vi "Quaternary_Layer.vi"(2 "Debug Mode":bool, 3 "Elapsed Time (s)":dbl, 4 "State":enum16{"Edit", "Start", "Run", "End", "Idle"}(ring), 5 "Argument List In":string[](array[string])) -> (0 "Status Out":string, 1 "Argument List Out":string[](array[string]))   [LabVIEW 2011]
panel:
  in  "PH3 run":bool
  in  "AsH3 run":bool
  in  "In run":bool
  in  "Ga run":bool
  in  "PH3 Flow":dbl
  in  "AsH3 Flow":dbl
  in  "In Flow":dbl
  in  "Ga Flow":dbl
  in  "Cancel":bool
  in  "OK":bool
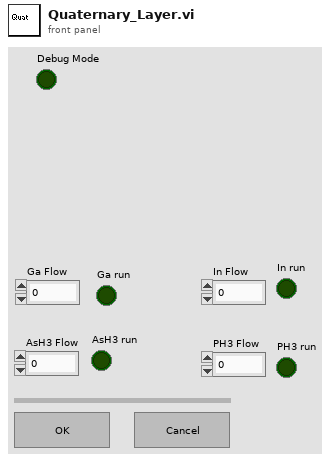
[diagram p1: front panel]
types:
  T1 = enum16{"Discrete", "Continuous", "Instantaneous"}
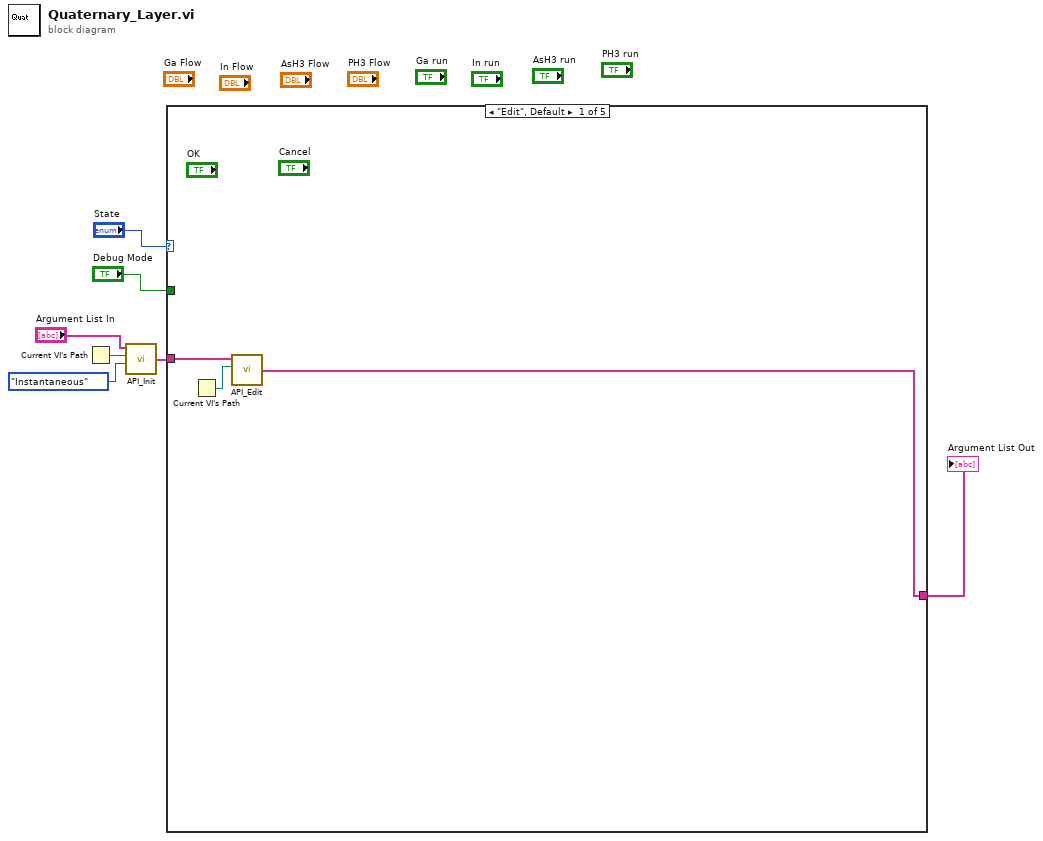
[diagram p0: block diagram]
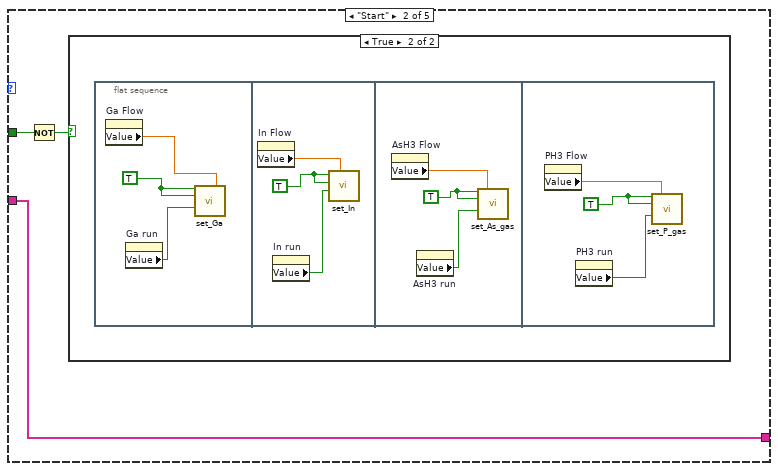
[diagram p2: hidden frame]
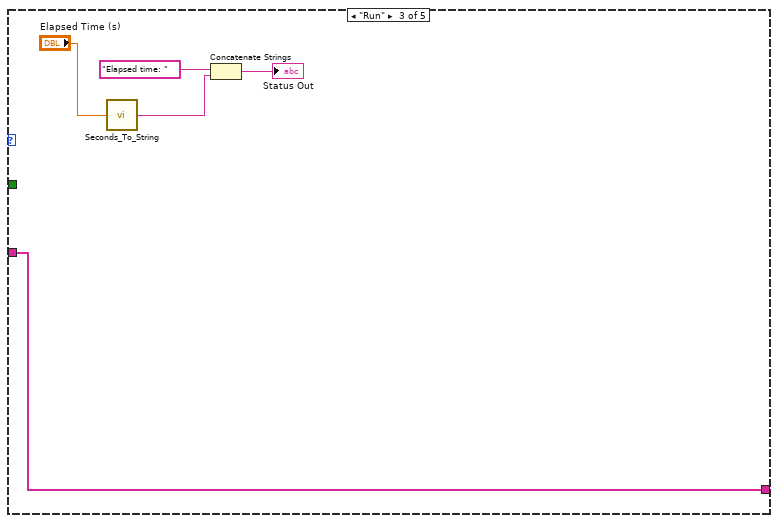
[diagram p4: hidden frame]
diagram:
  n1 = Current VI's Path() -> (path=w4:path)
  n2 = call "API_Init.vi"("API Mode"=T1."Instantaneous", "VI Path"=w4, "Argument List In"="Argument List In") -> ("Argument List Out"=w3:string[])  [unwired: 1 in]
  n3 = case shown="\"Edit\", Default" "State" {
    tunnel: [w8 w13 w26 w31 w32] -> w6
    tunnel: w3 -> [w9 w13 w26 w31 w32]
    tunnel: "Debug Mode" -> [_ w12 _ _ _]
    frame "Edit", Default {
      n4 = Current VI's Path() -> (path=w10:path)
      n5 = call "API_Edit.vi"("VI Path"=w10, "Argument List In"=w9) -> ("Argument List Out"=w8:string[])  [unwired: 2 in]
    }
    frame "Start" {
      n6 = Not(x=w12) -> (.not. x?=w11:bool)
      n7 = case shown="True" w11 {
        frame False {
        }
        frame True {
          n8 = flat-sequence {
            frame #0 {
              w16 = TRUE ("Ga Active")
              n9 = property on="Ga Flow" class="DigNum (strict)"() -> ("Value"=w15:dbl)  [unwired: 2 in, 2 out]
              n10 = property on="Ga run" class="Bool (strict)"() -> ("Value"=w14:bool)  [unwired: 2 in, 2 out]
              n11 = call "set_Ga.vi"("Ga Active"=w16, "Ga Flow 1"=w15, "Ga Bubbler"=w16, "Ga Run"=w14) -> ()  [unwired: 4 in, 8 out]
            }
            frame #1 {
              w19 = TRUE ("Ga Active")
              n12 = property on="In Flow" class="DigNum (strict)"() -> ("Value"=w18:dbl)  [unwired: 2 in, 2 out]
              n13 = property on="In run" class="Bool (strict)"() -> ("Value"=w17:bool)  [unwired: 2 in, 2 out]
              n14 = call "set_In.vi"("Indium Flow"=w18, "In Run"=w17, "In Bubbler"=w19, "In Active"=w19) -> ()  [unwired: 1 in, 5 out]
            }
            frame #2 {
              w21 = TRUE ("Ga Active")
              n15 = property on="AsH3 Flow" class="DigNum (strict)"() -> ("Value"=w22:dbl)  [unwired: 2 in, 2 out]
              n16 = property on="AsH3 run" class="Bool (strict)"() -> ("Value"=w20:bool)  [unwired: 2 in, 2 out]
              n17 = call "set_As_gas.vi"("As_Gas Active"=w21, "As_Gas Flow"=w22, "As_Gas In"=w21, "As_Gas Run"=w20) -> ()  [unwired: 2 in, 10 out]
            }
            frame #3 {
              w25 = TRUE ("Ga Active")
              n18 = property on="PH3 Flow" class="DigNum (strict)"() -> ("Value"=w24:dbl)  [unwired: 2 in, 2 out]
              n19 = property on="PH3 run" class="Bool (strict)"() -> ("Value"=w23:bool)  [unwired: 2 in, 2 out]
              n20 = call "set_P_gas.vi"("P_Gas Active"=w25, "P_Gas Flow"=w24, "P_Gas In"=w25, "P_Gas Run"=w23) -> ()  [unwired: 2 in, 10 out]
            }
          }
        }
      }
    }
    frame "Run" {
      n21 = call "Seconds_To_String.vi"("Seconds"="Elapsed Time (s)") -> ("Output String"=w28:string)
      n22 = Concatenate Strings("Elapsed time: " ("string"), w28) -> (→"Status Out":string)
    }
    frame "End" {
    }
    frame "Idle" {
    }
  }
  "Argument List Out" <- w6
